vi "Teleop.vi"(10 "Match Info":T1={"Autonomous Elapsed Seconds"=0.0, "TeleOp Elapsed Seconds"=0.0, "Disabled Elapsed Seconds"=0.0, "Visited Autonomous"=FALSE, "Visited TeleOp"=FALSE, "Visited Disabled"=FALSE, "Autonomous Settings"={"Autonomous Style"=enum."Independent", "VI Refnum"=refnum}}, 11 "Call Context":T2) -> ()   [LabVIEW 2014]
doc: "This VI is called for each TeleOp packet received from the DS where the robot is not disabled. It is often used to read from the joysticks and update I/O or to update setpoints for timed control loops. It should complete and return within 20 milliseconds or it may miss DS packets."
uses:
  <vilib>/Rock Robotics/WPI/DriverStation/WPI_DriverStationDerivedRobotMode.ctl
  <vilib>/Rock Robotics/WPI/DriverStation/WPI_DriverStationMatch Info.ctl
  <vilib>/Rock Robotics/Network Tables/SD Read Boolean.vi
  <vilib>/Rock Robotics/Network Tables/SD Read Number.vi
  <vilib>/Rock Robotics/WPI/Joystick/WPI_JoystickGetSetRefNum.vi
  <vilib>/Rock Robotics/WPI/RobotDrive/WPI_RobotDriveGetSetRefNum.vi
  <vilib>/Rock Robotics/WPI/RobotDrive/WPI_RobotDriveMecanumDrive_Polar.vi
  <vilib>/Rock Robotics/WPI/Solenoid/WPI_SolenoidSetEnum.vi
panel:
  out "Sample Slider 0":dbl(slide) scale=0.0..5.0
  out "Sample Boolean 1":bool
  out "Sample Boolean 0":bool
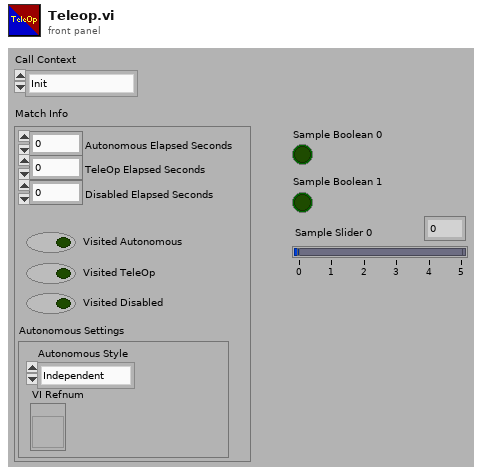
[diagram p1: front panel]
types:
  T1 = typedef "WPI_DriverStationMatch Info.ctl" = cluster{"Autonomous Elapsed Seconds":dbl, "TeleOp Elapsed Seconds":dbl, "Disabled Elapsed Seconds":dbl, "Visited Autonomous":bool, "Visited TeleOp":bool, "Visited Disabled":bool, "Autonomous Settings":cluster{"Autonomous Style":enum16{"Iterative", "Independent"}, "VI Refnum":refnum<vi>}}
  T2 = typedef "WPI_DriverStationDerivedRobotMode.ctl" = enum16{"Init", "Execute", "Stop"}
  T3 = typedef "WPI_JoystickDevRef.ctl" = cluster{"Device":T4}
  T4 = typedef "WPI_JoystickDeviceEnum.ctl" = enum16{"USB 0", "USB 1", "USB 2", "USB 3", "USB 4", "USB 5"}
  T5 = typedef "Joystick Buttons typedef.ctl" = cluster{"A":bool, "B":bool, "X":bool, "Y":bool, "Left bumper":bool, "Right bumper":bool, "Select":bool, "Start":bool}
  T6 = typedef "Joystick Axis typedefs.ctl" = cluster{"Left stick X":dbl, "Left stick Y":dbl, "Right stick X ":dbl, "Right stick Y":dbl, "Trigger":dbl}
  T7 = typedef "WPI_PotentiometerDevRef.ctl" = cluster{"DevStatus":errorcluster, "Controller":T8, "Analog Channel":T9, "Invert Output":bool}
  T8 = typedef "FPGA_TypedefAnalogModule.ctl" = enum16{"Controller 1"}
  T9 = typedef "FPGA_AIChannel.ctl" = enum8{"AI 0", "AI 1", "AI 2", "AI 3", "AI MXP 0", "AI MXP 1", "AI MXP 2", "AI MXP 3", "Invalid"}
  T10 = typedef "WPI_GyroDevRef.ctl" = cluster{"DevStatus":errorcluster, "Analog Module":T8, "Analog Channel":T9, "Offset":dbl, "Gain (VoltsPerDegree/Second)":dbl}
  T11 = typedef "WPI_SolenoidValue.ctl" = enum16{"Off", "On", "Forward", "Reverse"}
  T12 = typedef "WPI_RobotDriveDevRef.ctl" = cluster{"DevStatus":errorcluster, "Motors[]":T13[], "Square Inputs":bool, "Max Output":dbl}
  T13 = typedef "WPI_MotorControlDeviceRef.ctl" = cluster{"DeviceStatus":errorcluster, "Type":T14, "PWM":cluster{"Controller":T15, "PWM Channel":T16, "DeadBand":T17}, "CAN":cluster{"Device Number":u8, "Control Mode":T18, "Semaphore":T19, "Max Vout":dbl, "TalonSRX Control Mode":T20}, "Invert":bool, "TransformRef":T21, "InvTransformRef":T21}
  T14 = typedef "WPI_MotorControlType.ctl" = enum16{"PWM", "CAN", "CANTalonSRX"}
  T15 = typedef "FPGA_TypedefDigitalModule.ctl" = enum16{"Controller 1"}
  T16 = typedef "FPGA_DIOPWMChannel.ctl" = enum8{"PWM 0", "PWM 1", "PWM 2", "PWM 3", "PWM 4", "PWM 5", "PWM 6", "PWM 7", "PWM 8", "PWM 9", "PWM MXP 0", "PWM MXP 1", "PWM MXP 2", "PWM MXP 3", "PWM MXP 4", "PWM MXP 5", "PWM MXP 6", "PWM MXP 7", "PWM MXP 8", "PWM MXP 9", "Invalid"}
  T17 = typedef "WPI_PWMDeadband.ctl" = cluster{"Name":string, "maxPositivePwm":i32, "minPositivePwm":i32, "centerPwm":i32, "maxNegativePwm":i32, "minNegativePwm":i32, "angularRange":u16}
  T18 = typedef "WPI_CANJaguar_ControlMode.ctl" = enum8{"Percent VBus", "Current", "Speed", "Position", "Voltage"}
  T19 = typedef "Semaphore RefNum" = refnum<k1>
  T20 = typedef "WPI_CANTalonSRX_APIControlMode.ctl" = enum8{"Percent VBus", "Speed", "Position", "Slave", "Unchanged / Invalid"}
  T21 = typedef "WPI_PWMTransform_ConPane.ctl" = refnum<vi>
  T22 = typedef "WPI_SolenoidDevRef.ctl" = cluster{"DevStatus":errorcluster, "Pneumatics Control Module":u8, "Forward Solenoid Channel":T23, "Reverse Solenoid Channel":T23}
  T23 = typedef "WPI_SolenoidChannel.ctl" = enum8{"Solenoid 0", "Solenoid 1", "Solenoid 2", "Solenoid 3", "Solenoid 4", "Solenoid 5", "Solenoid 6", "Solenoid 7", "Invalid"}
  T24 = typedef "WPI_SwitchDevRef.ctl" = cluster{"DevStatus":errorcluster, "DIO Channel":T25, "Controller":T15, "CntIndex":T26, "Normally Closed":bool}
  T25 = typedef "FPGA_DIOChannel.ctl" = enum8{"DIO 0", "DIO 1", "DIO 2", "DIO 3", "DIO 4", "DIO 5", "DIO 6", "DIO 7", "DIO 8", "DIO 9", "DIO MXP 0", "DIO MXP 1", "DIO MXP 2", "DIO MXP 3", "DIO MXP 4", "DIO MXP 5", "DIO MXP 6", "DIO MXP 7", "DIO MXP 8", "DIO MXP 9", "DIO MXP 10", "DIO MXP 11", "DIO MXP 12", "DIO MXP 13", "DIO MXP 14", "DIO MXP 15", "Invalid"}
  T26 = typedef "FPGA_CounterCtrSystemIndex.ctl" = enum8{"Ctr 0", "Ctr 1", "Ctr 2", "Ctr 3", "Ctr 4", "Ctr 5", "Ctr 6", "Ctr 7", "Invalid"}
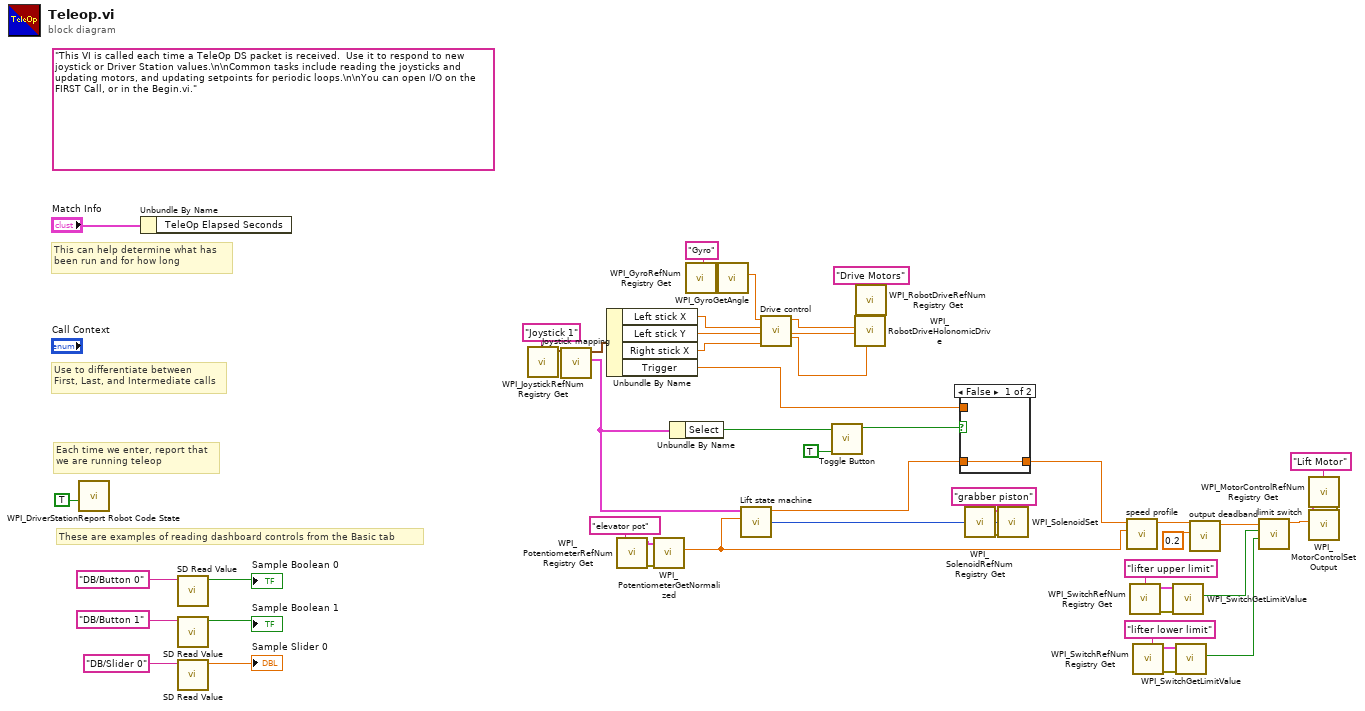
[diagram p0: block diagram]
diagram:
  (unwired) "This VI is called each time a TeleOp DS packet is received.  Use it to respond to new joystick or Driver Station values.\n\nCommon tasks include reading the joysticks and updating motors, and updating setpoints for periodic loops.\n\nYou can open I/O on the FIRST Call, or in the Begin.vi."
  # "These are examples of reading dashboard controls from the Basic tab"
  # "Each time we enter, report that\nwe are running teleop"
  # "Use to differentiate between\nFirst, Last, and Intermediate calls"
  # "This can help determine what has\nbeen run and for how long"
  n1 = call <vilib>:"WPI_DriverStationReport Robot Code State.vi"("TeleOp"=TRUE ("Autonomous")) -> ()  [unwired: 10 in, 1 out]
  n2 = Unbundle By Name("Match Info") -> ()  [unwired: 1 out]
  n3 = call-poly <vilib>:"SD Read Value.vi"("Name"="DB/Button 0" ("refnum name")) -> ("Boolean"=→"Sample Boolean 0":bool)  [unwired: 8 in, 2 out]
  n4 = call-poly <vilib>:"SD Read Value.vi"("Name"="DB/Button 1" ("refnum name")) -> ("Boolean"=→"Sample Boolean 1":bool)  [unwired: 8 in, 2 out]
  n5 = call-poly <vilib>:"SD Read Value.vi"("Name"="DB/Slider 0" ("refnum name")) -> ("Numeric"=→"Sample Slider 0":dbl)  [unwired: 8 in, 2 out]
  n6 = call <vilib>:"WPI_JoystickRefNum Registry Get.vi"("refnum name"="Joystick 1") -> ("JoystickDevRef"=w45:T3)  [unwired: 9 in, 1 out]
  n7 = call "Joystick mapping.vi"("JoystickDevRef"=w45) -> ("Joystick Buttons"=w18:T5, "Joystick Axis"=w41:T6)  [unwired: 9 in]
  n8 = Unbundle By Name(w41) -> ("Left stick X"=w2:dbl, "Left stick Y"=w3:dbl, "Right stick X"=w4:dbl, "Trigger"=w17:dbl)
  n9 = call <vilib>:"WPI_PotentiometerRefNum Registry Get.vi"("refnum name"="elevator pot") -> ("error out"=w34:errorcluster, "PotDevRef"=w33:T7)  [unwired: 9 in]
  n10 = call <vilib>:"WPI_PotentiometerGetNormalized.vi"("error in"=w34, "PotDevRef"=w33) -> ("Normalized Value"=w15:dbl)  [unwired: 7 in, 2 out]
  n11 = Unbundle By Name(w18) -> ("Select"=w7:bool)
  n12 = call <vilib>:"WPI_GyroRefNum Registry Get.vi"("refnum name"="Gyro") -> ("error out"=w40:errorcluster, "GyroDevRef"=w39:T10)  [unwired: 9 in]
  n13 = call <vilib>:"WPI_GyroGetAngle.vi"("error in (no error)"=w40, "GyroDevRef"=w39) -> ("Angle"=w1:dbl)  [unwired: 6 in, 3 out]
  n14 = call "Lift state machine.vi"("Grabber Height"=w15, "Joystick Buttons"=w18) -> ("Value"=w11:T11, "Motor speed"=w28:dbl)  [unwired: 8 in]
  n15 = call "Drive control.vi"("Right stick X"=w4, "Left stick Y"=w3, "Left stick X"=w2, "Gyro angle"=w1) -> ("Rotation"=w35:dbl, "Direction"=w36:dbl, "Magnitude"=w37:dbl)  [unwired: 5 in]
  n16 = call "Toggle Button.vi"("starting state"=TRUE, "toggle button"=w7) -> ("button toggled value"=w5:bool)  [unwired: 9 in]
  n17 = call <vilib>:"WPI_RobotDriveRefNum Registry Get.vi"("refnum name"="Drive Motors") -> ("error out"=w44:errorcluster, "RobotDriveDevRef"=w43:T12)  [unwired: 9 in]
  n18 = call-poly <vilib>:"WPI_RobotDriveHolonomicDrive.vi"("Rotation"=w35, "error in (no error)"=w44, "Direction"=w36, "Magnitude"=w37, "RobotDriveDevRef"=w43) -> ()  [unwired: 4 in, 3 out]
  n19 = case shown="False" w5 {
    tunnel: [w55 w56] -> w16
    tunnel: w28 -> [w55 _]
    tunnel: w17 -> [_ w56]
    frame False {
    }
    frame True {
    }
  }
  n20 = call <vilib>:"WPI_SolenoidRefNum Registry Get.vi"("refnum name"="grabber piston") -> ("error out"=w13:errorcluster, "SolenoidDevRef"=w14:T22)  [unwired: 9 in]
  n21 = call-poly <vilib>:"WPI_SolenoidSet.vi"("error in (no error)"=w13, "Value"=w11, "SolenoidDevRef"=w14) -> ()  [unwired: 7 in, 2 out]
  n22 = call "speed profile.vi"("Pot position"=w15, "motor speed"=w16) -> ("motor output"=w10:dbl)  [unwired: 9 in]
  n23 = call <vilib>:"WPI_SwitchRefNum Registry Get.vi"("refnum name"="lifter upper limit") -> ("error out"=w21:errorcluster, "SwitchDevRef"=w26:T24)  [unwired: 9 in]
  n24 = call <vilib>:"WPI_SwitchRefNum Registry Get.vi"("refnum name"="lifter lower limit") -> ("error out"=w22:errorcluster, "SwitchDevRef"=w25:T24)  [unwired: 9 in]
  n25 = call <vilib>:"WPI_SwitchGetLimitValue.vi"("error in (no error)"=w21, "SwitchDevRef"=w26) -> ("Switch Pressed"=w20:bool)  [unwired: 7 in, 2 out]
  n26 = call <vilib>:"WPI_SwitchGetLimitValue.vi"("error in (no error)"=w22, "SwitchDevRef"=w25) -> ("Switch Pressed"=w19:bool)  [unwired: 7 in, 2 out]
  n27 = call "output deadband.vi"("deadband width"=0.2, "motor input"=w10) -> ("motor output"=w9:dbl)  [unwired: 9 in]
  n28 = call "limit switch.vi"("lower limit"=w19, "upper limit"=w20, "motor input"=w9) -> ("motor output"=w27:dbl)  [unwired: 8 in]
  n29 = call <vilib>:"WPI_MotorControlRefNum Registry Get.vi"("refnum name"="Lift Motor") -> ("error out"=w29:errorcluster, "MotorControlDevRef"=w30:T13)  [unwired: 9 in]
  n30 = call <vilib>:"WPI_MotorControlSetOutput.vi"("error in (no error)"=w29, "Output"=w27, "MotorControlDevRef"=w30) -> ()  [unwired: 6 in, 3 out]
